vi "Get_Set_Statistics2.vi"(6 "Get/Set":T2, 8 "Status/Errors in":refnum<vi>, 9 "Page Statistics 2":refnum<vi>, 10 "Time window":dbl, 11 "Page Statistics 2 in":T1 {"Time_difference_zoom_count" format="%#.9f"; "Time difference overshoot" format="%#_2f"; "Data points overshoot" format="%#_2f"; "St.Dev.overshoot" format="%#_2f"; "Baseline_overshoot" format="%#_2f"}) -> (0 "Status/Errors out":refnum<vi>, 1 "Page Statistics 2":refnum<vi>, 3 "Page Statistics 2 out":T1 {"Time_difference_zoom_count" format="%#.9f"; "Time difference overshoot" format="%#_2f"; "Data points overshoot" format="%#_2f"; "St.Dev.overshoot" format="%#_2f"; "Baseline_overshoot" format="%#_2f"})   [LabVIEW 2010]
uses:
  Controls/TabPage_Statistics2.ctl
  Controls/Get_Set_Statistics_Options2.ctl
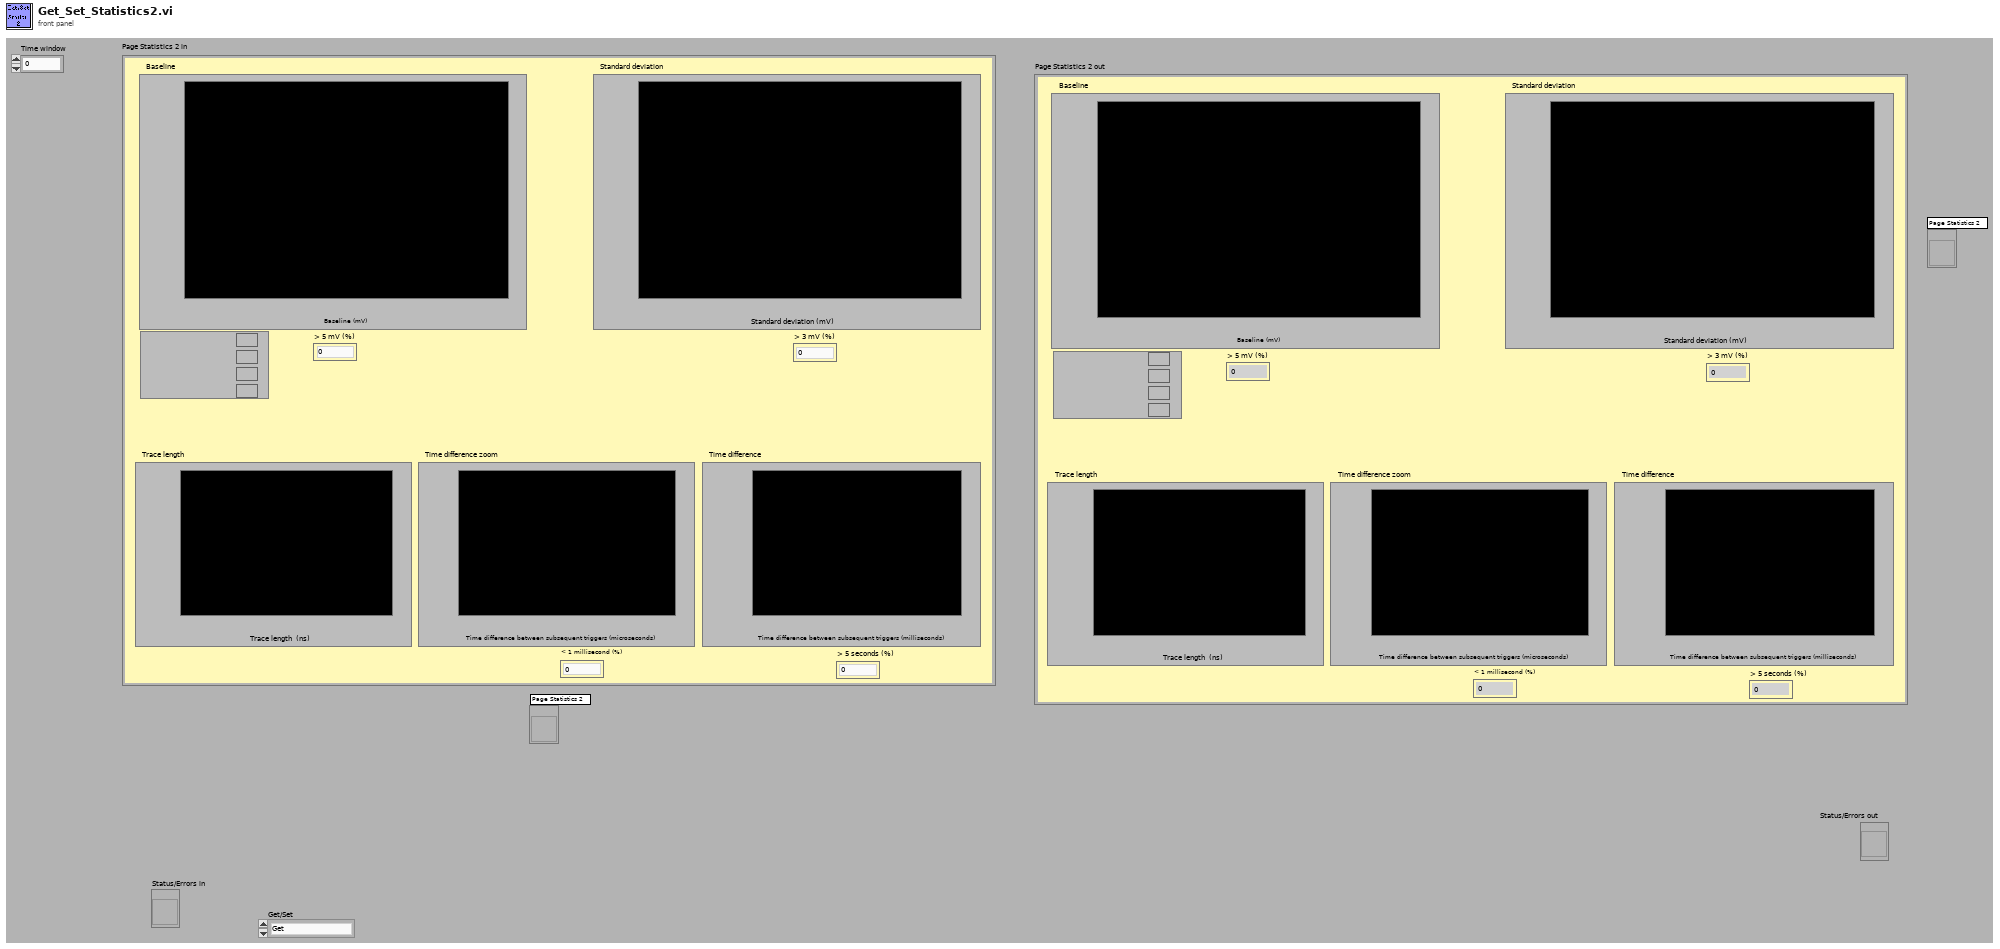
[diagram p1: front panel]
types:
  T1 = typedef "TabPage_Statistics2.ctl" = cluster{"Baseline_overshoot":dbl, "St.Dev.overshoot":dbl, "Data points overshoot":dbl, "Time difference overshoot":dbl, "Time_difference_zoom_count":dbl, "Baseline.His":cluster{"t0":i32, "dt":i32, "Histogram":i32[][]}, "St._dev.His":cluster{"t0":i32, "dt":i32, "Histogram":i32[][]}, "Trace_length.His":cluster{"t0":i32, "dt":i32, "Histogram":i32[][]}, "Time_difference.His_zoom":cluster{"t0":i32, "dt":i32, "Histogram":i32[][]}, "Time_difference.His":cluster{"t0":i32, "dt":i32, "Histogram":i32[][]}, "Baselin Entries":u64, "Baseline Overshoots":u64, "Time Entries ":u64, "Time  Overshoots ":u64, "St.dev. Entries ":u64, "St.dev.  Overshoots ":u64, "Length  Entries ":u64, "Length Overshoots ":u64, "Time zoom Entries ":u64, "Time zoom Overshoots ":u64}
  T2 = typedef "Get_Set_Statistics_Options2.ctl" = enum16{"Get", "Set"}
  T3 = cluster{"Baseline_overshoot":dbl, "St.Dev.overshoot":dbl, "Data points overshoot":dbl, "Time difference overshoot":dbl, "Time_difference_zoom_count":dbl, "Baseline.His":cluster{"t0":i32, "dt":i32, "Histogram":i32[][]}, "St._dev.His":cluster{"t0":i32, "dt":i32, "Histogram":i32[][]}, "Trace_length.His":cluster{"t0":i32, "dt":i32, "Histogram":i32[][]}, "Time_difference.His_zoom":cluster{"t0":i32, "dt":i32, "Histogram":i32[][]}, "Time_difference.His":cluster{"t0":i32, "dt":i32, "Histogram":i32[][]}, "Baselin Entries":u64, "Baseline Overshoots":u64, "Time Entries":u64, "Time  Overshoots":u64, "St.dev. Entries":u64, "St.dev.  Overshoots":u64, "Length  Entries":u64, "Length Overshoots":u64, "Time zoom Entries":u64, "Time zoom Overshoots":u64}
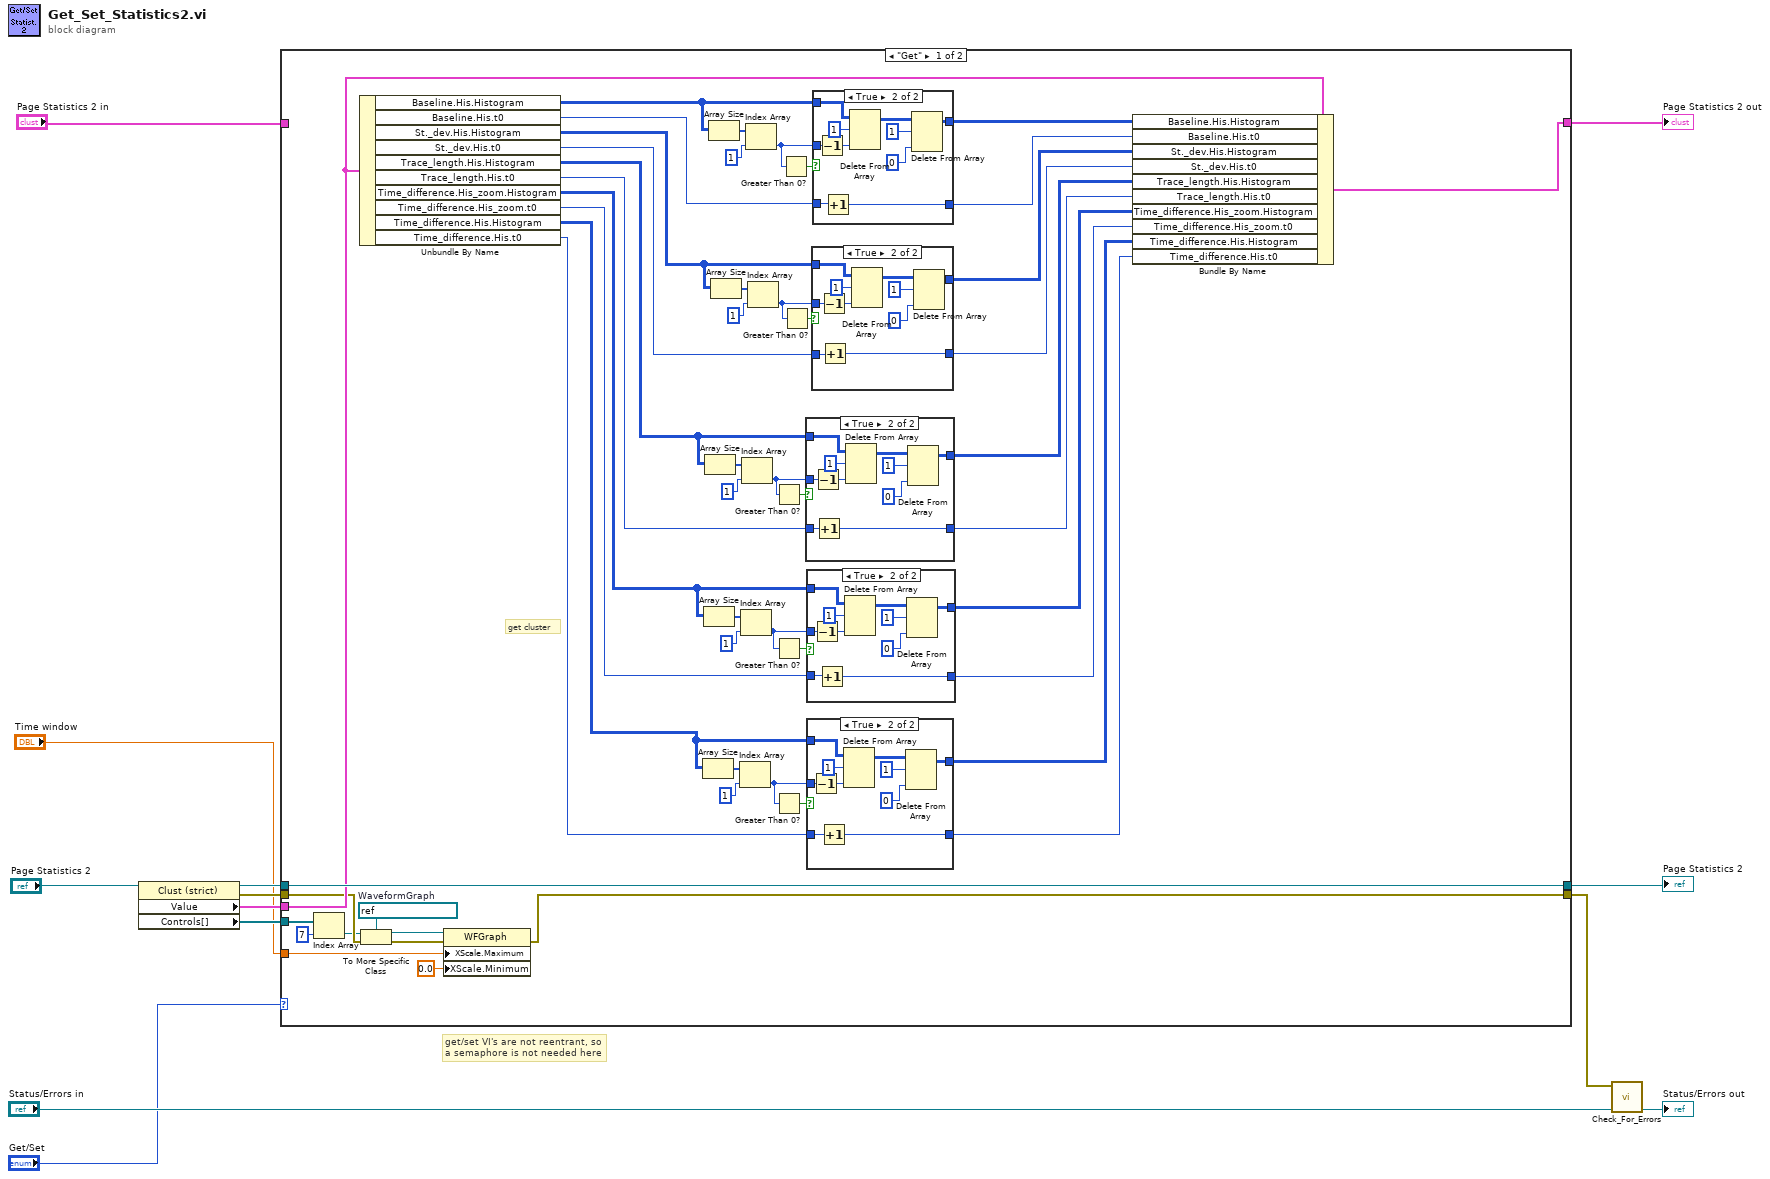
[diagram p0: block diagram]
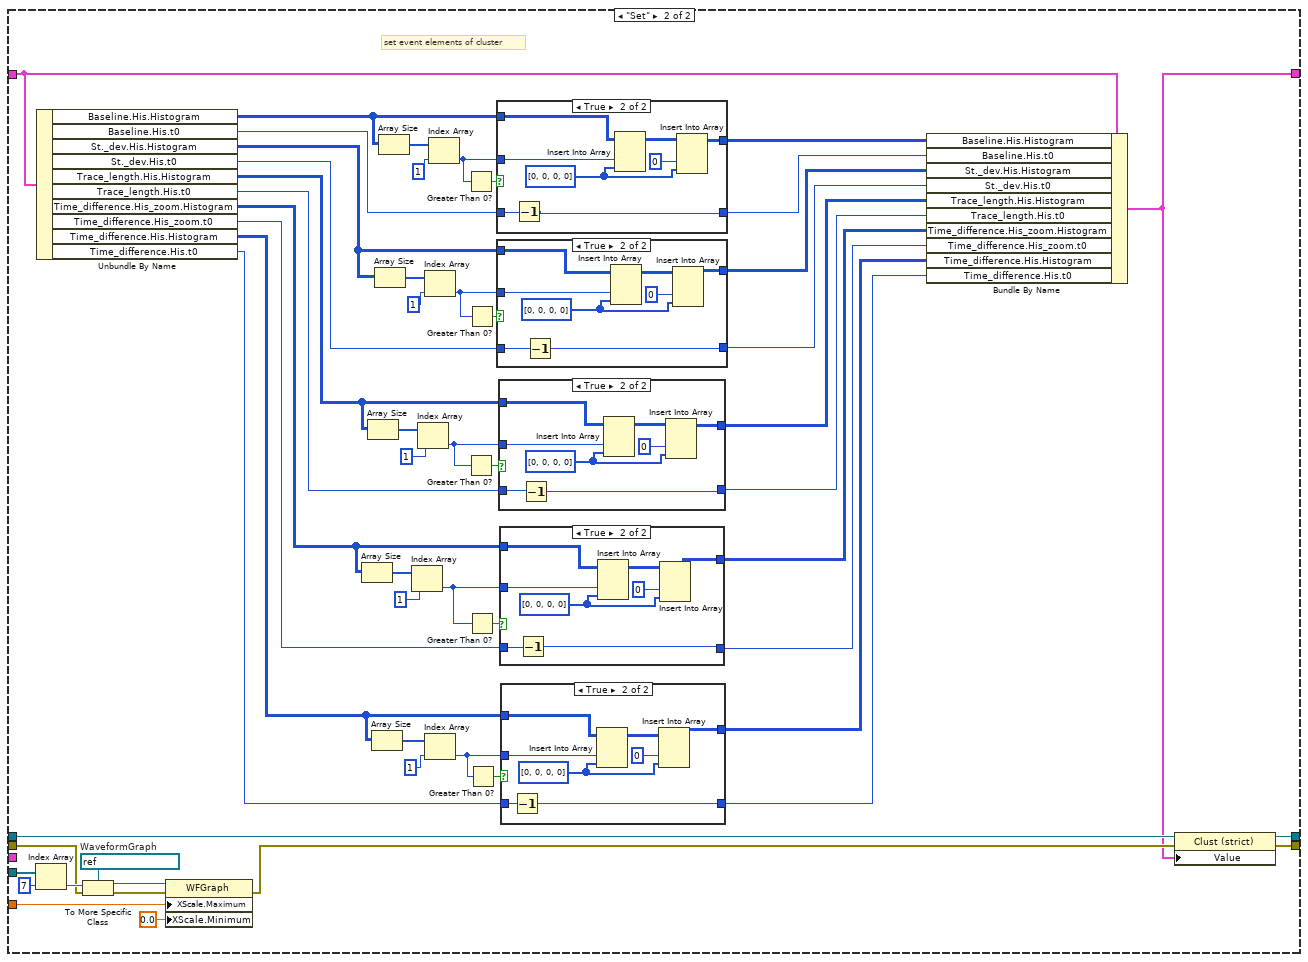
[diagram p7: hidden frame]
diagram:
  # "get/set VI's are not reentrant, so\na semaphore is not needed here"
  n1 = property class="Clust (strict)"(reference="Page Statistics 2") -> (reference out=w10:refnum<vi>, error out=w9:errorcluster, "Value"=w8:T3, "Controls[]"=w2:refnum<vi>[])  [unwired: 1 in]
  n2 = case shown="\"Get\"" "Get/Set" {
    tunnel: "Page Statistics 2 in" -> [_ w166]
    tunnel: w10 -> [w66 w181]
    tunnel: [w66 w179] -> w4
    tunnel: [w16 w180] -> w12
    tunnel: [w60 w164] -> w3
    tunnel: w8 -> [w61 _]
    tunnel: w9 -> [w17 w172]
    tunnel: w2 -> [w14 w178]
    tunnel: "Time window" -> [w18 w170]
    frame "Get" {
      w22 = refnum<vi> refnum  # WaveformGraph
      # "get cluster"
      n3 = Index Array(array=w14, index=7) -> (element=w15:refnum<vi>)
      n4 = Unbundle By Name(w61) -> ("Baseline.His.Histogram"=w63:i32[][], "Baseline.His.t0"=w33:i32, "St._dev.His.Histogram"=w53:i32[][], "St._dev.His.t0"=w32:i32, "Trace_length.His.Histogram"=w52:i32[][], "Trace_length.His.t0"=w31:i32, "Time_difference.His_zoom.Histogram"=w51:i32[][], "Time_difference.His_zoom.t0"=w30:i32, "Time_difference.His.Histogram"=w45:i32[][], "Time_difference.His.t0"=w29:i32)
      n5 = To More Specific Class(target class=w22, reference=w15, error in=w17) -> (specific class reference=w21:refnum<vi>, error out=w20:errorcluster)
      n6 = property class="WFGraph"(reference=w21, error in=w20, "XScale.Maximum"=w18, "XScale.Minimum"=0.0 ("X Scale.Range:Minimum")) -> (error out=w16:errorcluster)  [unwired: 1 out]
      n7 = Array Size(array=w45) -> (size(s)=w47:i32[])
      n8 = Array Size(array=w51) -> (size(s)=w55:i32[])
      n9 = Array Size(array=w52) -> (size(s)=w57:i32[])
      n10 = Array Size(array=w63) -> (size(s)=w65:i32[])
      n11 = Array Size(array=w53) -> (size(s)=w59:i32[])
      n12 = Index Array(array=w47, index=1) -> (element=w34:i32)
      n13 = Index Array(array=w55, index=1) -> (element=w37:i32)
      n14 = Index Array(array=w57, index=1) -> (element=w39:i32)
      n15 = Index Array(array=w65, index=1) -> (element=w42:i32)
      n16 = Index Array(array=w59, index=1) -> (element=w40:i32)
      n17 = Greater Than 0?(x=w39) -> (x > 0?=w38:bool)
      n18 = Greater Than 0?(x=w37) -> (x > 0?=w36:bool)
      n19 = Greater Than 0?(x=w34) -> (x > 0?=w35:bool)
      n20 = Greater Than 0?(x=w42) -> (x > 0?=w43:bool)
      n21 = Greater Than 0?(x=w40) -> (x > 0?=w41:bool)
      n22 = case shown="True" w38 {
        tunnel: w39 -> [_ w97]
        tunnel: w52 -> [w92 w96]
        tunnel: [w92 w95] -> w49
        tunnel: w31 -> [w91 w94]
        tunnel: [w91 w93] -> w26
        frame False {
        }
        frame True {
          n23 = Decrement(x=w97) -> (x-1=w98:i32)
          n24 = Increment(x=w94) -> (x+1=w93:i32)
          n25 = Delete From Array(array=w96, length=1, index (col)=w98) -> (array with subset deleted=w102:i32[][])  [unwired: 1 in, 1 out]
          n26 = Delete From Array(array=w102, length=1 ("disabled index (col)"), index (col)=0 ("disabled index (col)")) -> (array with subset deleted=w95:i32[][])  [unwired: 1 in, 1 out]
        }
      }
      n27 = case shown="True" w36 {
        tunnel: w37 -> [_ w85]
        tunnel: w51 -> [w80 w84]
        tunnel: [w80 w83] -> w48
        tunnel: w30 -> [w79 w82]
        tunnel: [w79 w81] -> w25
        frame False {
        }
        frame True {
          n28 = Decrement(x=w85) -> (x-1=w86:i32)
          n29 = Increment(x=w82) -> (x+1=w81:i32)
          n30 = Delete From Array(array=w84, length=1, index (col)=w86) -> (array with subset deleted=w90:i32[][])  [unwired: 1 in, 1 out]
          n31 = Delete From Array(array=w90, length=1 ("disabled index (col)"), index (col)=0 ("disabled index (col)")) -> (array with subset deleted=w83:i32[][])  [unwired: 1 in, 1 out]
        }
      }
      n32 = case shown="True" w35 {
        tunnel: w34 -> [_ w73]
        tunnel: w45 -> [w68 w72]
        tunnel: [w68 w71] -> w44
        tunnel: w29 -> [w67 w70]
        tunnel: [w67 w69] -> w24
        frame False {
        }
        frame True {
          n33 = Decrement(x=w73) -> (x-1=w74:i32)
          n34 = Increment(x=w70) -> (x+1=w69:i32)
          n35 = Delete From Array(array=w72, length=1, index (col)=w74) -> (array with subset deleted=w78:i32[][])  [unwired: 1 in, 1 out]
          n36 = Delete From Array(array=w78, length=1 ("disabled index (col)"), index (col)=0 ("disabled index (col)")) -> (array with subset deleted=w71:i32[][])  [unwired: 1 in, 1 out]
        }
      }
      n37 = case shown="True" w41 {
        tunnel: w40 -> [_ w109]
        tunnel: w53 -> [w104 w108]
        tunnel: [w104 w107] -> w50
        tunnel: w32 -> [w103 w106]
        tunnel: [w103 w105] -> w27
        frame False {
        }
        frame True {
          n38 = Decrement(x=w109) -> (x-1=w110:i32)
          n39 = Increment(x=w106) -> (x+1=w105:i32)
          n40 = Delete From Array(array=w108, length=1, index (col)=w110) -> (array with subset deleted=w114:i32[][])  [unwired: 1 in, 1 out]
          n41 = Delete From Array(array=w114, length=1 ("disabled index (col)"), index (col)=0 ("disabled index (col)")) -> (array with subset deleted=w107:i32[][])  [unwired: 1 in, 1 out]
        }
      }
      n42 = case shown="True" w43 {
        tunnel: w63 -> [w116 w126]
        tunnel: [w116 w123] -> w62
        tunnel: w42 -> [_ w119]
        tunnel: w33 -> [w115 w118]
        tunnel: [w115 w117] -> w28
        frame False {
        }
        frame True {
          n43 = Decrement(x=w119) -> (x-1=w120:i32)
          n44 = Increment(x=w118) -> (x+1=w117:i32)
          n45 = Delete From Array(array=w126, length=1, index (col)=w120) -> (array with subset deleted=w125:i32[][])  [unwired: 1 in, 1 out]
          n46 = Delete From Array(array=w125, length=1 ("disabled index (col)"), index (col)=0 ("disabled index (col)")) -> (array with subset deleted=w123:i32[][])  [unwired: 1 in, 1 out]
        }
      }
      n47 = Bundle By Name(cluster=w61, "Baseline.His.Histogram"=w62, "Baseline.His.t0"=w28, "St._dev.His.Histogram"=w50, "St._dev.His.t0"=w27, "Trace_length.His.Histogram"=w49, "Trace_length.His.t0"=w26, "Time_difference.His_zoom.Histogram"=w48, "Time_difference.His_zoom.t0"=w25, "Time_difference.His.Histogram"=w44, "Time_difference.His.t0"=w24) -> (w60:T3)
    }
    frame "Set" {
      w175 = refnum<vi> refnum  # WaveformGraph
      # "set event elements of cluster"
      n48 = Index Array(array=w178, index=7) -> (element=w176:refnum<vi>)
      n49 = Unbundle By Name(w166) -> ("Baseline.His.Histogram"=w167:i32[][], "Baseline.His.t0"=w137:i32, "St._dev.His.Histogram"=w161:i32[][], "St._dev.His.t0"=w136:i32, "Trace_length.His.Histogram"=w156:i32[][], "Trace_length.His.t0"=w135:i32, "Time_difference.His_zoom.Histogram"=w152:i32[][], "Time_difference.His_zoom.t0"=w134:i32, "Time_difference.His.Histogram"=w148:i32[][], "Time_difference.His.t0"=w133:i32)
      n50 = To More Specific Class(target class=w175, reference=w176, error in=w172) -> (specific class reference=w174:refnum<vi>, error out=w173:errorcluster)
      n51 = property class="WFGraph"(reference=w174, error in=w173, "XScale.Maximum"=w170, "XScale.Minimum"=0.0 ("X Scale.Range:Minimum")) -> (error out=w171:errorcluster)  [unwired: 1 out]
      n52 = Array Size(array=w152) -> (size(s)=w155:i32[])
      n53 = Array Size(array=w156) -> (size(s)=w159:i32[])
      n54 = Array Size(array=w148) -> (size(s)=w151:i32[])
      n55 = Array Size(array=w161) -> (size(s)=w163:i32[])
      n56 = Array Size(array=w167) -> (size(s)=w169:i32[])
      n57 = Index Array(array=w155, index=1) -> (element=w143:i32)
      n58 = Index Array(array=w159, index=1) -> (element=w144:i32)
      n59 = Index Array(array=w163, index=1) -> (element=w140:i32)
      n60 = Index Array(array=w151, index=1) -> (element=w141:i32)
      n61 = Index Array(array=w169, index=1) -> (element=w146:i32)
      n62 = Greater Than 0?(x=w146) -> (x > 0?=w147:bool)
      n63 = Greater Than 0?(x=w144) -> (x > 0?=w145:bool)
      n64 = Greater Than 0?(x=w140) -> (x > 0?=w139:bool)
      n65 = Greater Than 0?(x=w143) -> (x > 0?=w142:bool)
      n66 = Greater Than 0?(x=w141) -> (x > 0?=w138:bool)
      n67 = case shown="True" w147 {
        tunnel: w167 -> [w223 w231]
        tunnel: [w223 w227] -> w165
        tunnel: w146 -> [_ w226]
        tunnel: w137 -> [w222 w225]
        tunnel: [w222 w224] -> w132
        frame False {
        }
        frame True {
          w228 = i32[] [0, 0, 0, 0] ("new element/subarray")
          n68 = Decrement(x=w225) -> (x-1=w224:i32)
          n69 = Insert Into Array(array=w231, index (col)=w226, new element=w228) -> (w230:i32[][])  [unwired: 1 in]
          n70 = Insert Into Array(array=w230, index (col)=0 ("disabled index (col)"), new element=w228) -> (w227:i32[][])  [unwired: 1 in]
        }
      }
      n71 = case shown="True" w139 {
        tunnel: w161 -> [w213 w218]
        tunnel: [w213 w217] -> w160
        tunnel: w140 -> [_ w216]
        tunnel: w136 -> [w212 w215]
        tunnel: [w212 w214] -> w131
        frame False {
        }
        frame True {
          w219 = i32[] [0, 0, 0, 0] ("new element/subarray")
          n72 = Decrement(x=w215) -> (x-1=w214:i32)
          n73 = Insert Into Array(array=w218, index (col)=w216, new element=w219) -> (w221:i32[][])  [unwired: 1 in]
          n74 = Insert Into Array(array=w221, index (col)=0 ("disabled index (col)"), new element=w219) -> (w217:i32[][])  [unwired: 1 in]
        }
      }
      n75 = case shown="True" w145 {
        tunnel: [w203 w208] -> w157
        tunnel: w156 -> [w203 w207]
        tunnel: w144 -> [_ w206]
        tunnel: w135 -> [w202 w205]
        tunnel: [w202 w204] -> w130
        frame False {
        }
        frame True {
          w209 = i32[] [0, 0, 0, 0] ("new element/subarray")
          n76 = Decrement(x=w205) -> (x-1=w204:i32)
          n77 = Insert Into Array(array=w207, index (col)=w206, new element=w209) -> (w211:i32[][])  [unwired: 1 in]
          n78 = Insert Into Array(array=w211, index (col)=0 ("disabled index (col)"), new element=w209) -> (w208:i32[][])  [unwired: 1 in]
        }
      }
      n79 = case shown="True" w142 {
        tunnel: [w193 w198] -> w153
        tunnel: w152 -> [w193 w197]
        tunnel: w143 -> [_ w196]
        tunnel: w134 -> [w192 w195]
        tunnel: [w192 w194] -> w129
        frame False {
        }
        frame True {
          w199 = i32[] [0, 0, 0, 0] ("new element/subarray")
          n80 = Decrement(x=w195) -> (x-1=w194:i32)
          n81 = Insert Into Array(array=w197, index (col)=w196, new element=w199) -> (w201:i32[][])  [unwired: 1 in]
          n82 = Insert Into Array(array=w201, index (col)=0 ("disabled index (col)"), new element=w199) -> (w198:i32[][])  [unwired: 1 in]
        }
      }
      n83 = case shown="True" w138 {
        tunnel: w141 -> [_ w188]
        tunnel: [w183 w187] -> w149
        tunnel: w148 -> [w183 w186]
        tunnel: w133 -> [w182 w185]
        tunnel: [w182 w184] -> w128
        frame False {
        }
        frame True {
          w189 = i32[] [0, 0, 0, 0] ("new element/subarray")
          n84 = Decrement(x=w185) -> (x-1=w184:i32)
          n85 = Insert Into Array(array=w186, index (col)=w188, new element=w189) -> (w191:i32[][])  [unwired: 1 in]
          n86 = Insert Into Array(array=w191, index (col)=0 ("disabled index (col)"), new element=w189) -> (w187:i32[][])  [unwired: 1 in]
        }
      }
      n87 = Bundle By Name(cluster=w166, "Baseline.His.Histogram"=w165, "Baseline.His.t0"=w132, "St._dev.His.Histogram"=w160, "St._dev.His.t0"=w131, "Trace_length.His.Histogram"=w157, "Trace_length.His.t0"=w130, "Time_difference.His_zoom.Histogram"=w153, "Time_difference.His_zoom.t0"=w129, "Time_difference.His.Histogram"=w149, "Time_difference.His.t0"=w128) -> (w164:T1)
      n88 = property class="Clust (strict)"(reference=w181, error in=w171, "Value"=w164) -> (reference out=w179:refnum<vi>, error out=w180:errorcluster)
    }
  }
  "Page Statistics 2" <- w4
  "Page Statistics 2 out" <- w3
  n89 = call "Check_For_Errors.vi"("Status/Errors in"="Status/Errors in", "error in"=w12) -> ("Status/Errors out"=→"Status/Errors out":refnum<vi>)  [unwired: 9 out]
